vi "GMLAN InitializeConnection.vi"(0 "CAN Interface":string(combo)="CAN1", 5 "Baudrate":u32, 7 "Transmit ID":u32, 9 "Receive ID":u32, 11 "error in (no error)":errorcluster, 12 "UUDT Receive ID":u32) -> (4 "UUDT Engine":T1, 6 "ADCS Ref":T2, 15 "error out":errorcluster)   [LabVIEW 2015, in "GMLAN.lvlib"]
uses:
  GMLAN.lvlib
  <vilib>/Automotive Diagnostic Command Set/Diagnostic Transport.llb/Diag Reference.ctl
  <vilib>/Automotive Diagnostic Command Set/Diagnostic Transport.llb/Transport Protocol Selector.ctl
  <vilib>/Automotive Diagnostic Command Set/Diagnostic Transport.llb/Diag CAN Frame Log.ctl
  _SubVIs/UUDT Engine Refs.ctl
  _SubVIs/UUDT Engine Connection List_Action.ctl
  <vilib>/xnet/xnet.llb/XNET Create Session (Frame Input Queued).vi
  <vilib>/addons/Automotive Diagnostic Command Set/NI_Automotive Diagnostic Command Set.lvlib
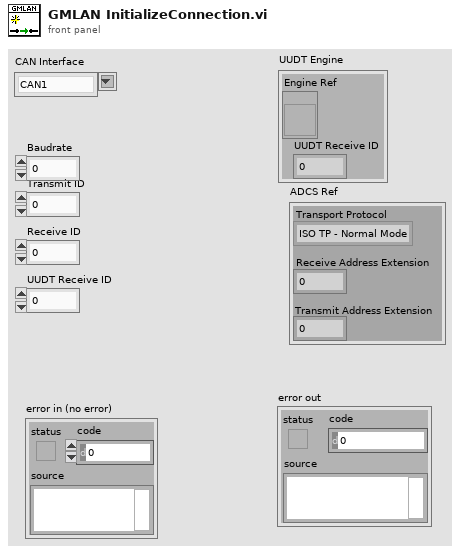
[diagram p1: front panel]
types:
  T1 = typedef "GMLAN.lvlib/UUDT Engine Refs.ctl" = cluster{"Engine Ref":refnum<vi>, "UUDT Receive ID":u32}
  T2 = typedef "NI_Automotive Diagnostic Command Set.lvlib/Diag Reference.ctl" = cluster{"Diag CAN Handle":u32, "Transport Protocol":T3, "Receive Address Extension":u8, "Transmit Address Extension":u8, "Receive CAN Id":u32, "Transmit CAN Id":u32, "Diag CAN Queue":refnum<queue>, "Log Frames ?":bool, "My TP Address":u8, "Other TP Address":u8, "T1":u16, "T2":u16, "T3":u16, "T4":u16, "Tx SN":u8, "Block Size":u8, "Rx SN":u8, "VW TP Initialized?":bool, "Tx block no":u8, "baud rate":u32, "Interface":string, "Channel Diag CAN Handle":u32, "UDP Connection ID":refnum<k16>, "TCP Connection ID":refnum<k5>, "Target IP Addr":u32, "Source Address":u16, "Target Address":u16, "Send Header NACK?":bool, "DLL Handle":u32, "NAD":u8, "Time Stamp read first":dbl, "Time Stamp read last":dbl, "Time Stamp write first":dbl, "Time Stamp write last":dbl, "Time Stamp write":dbl, "Time Stamp read":dbl}
  T3 = typedef "NI_Automotive Diagnostic Command Set.lvlib/Transport Protocol Selector.ctl" = enum16{"ISO TP - Normal Mode", "ISO TP - Mixed Mode", "VW TP 2.0", "Diagnostics on IP", "ISO TP LIN"}
  T4 = typedef "GMLAN.lvlib/UUDT Engine Connection List_Action.ctl" = enum8{"Initialize", "Write", "Add", "Read"}
  T5 = cluster{"Parameter Name":string, "Initial Settings":variant}
  T6 = cluster{"Frame name":string, "Identifier":u32, "Payload Length":u32, "Timing Type":u32, "Transmit Time":dbl, "Extended Identifier?":bool, "Comment":string}
  T7 = cluster{"Parameter Name":string, "Initial Settings":variant}[]
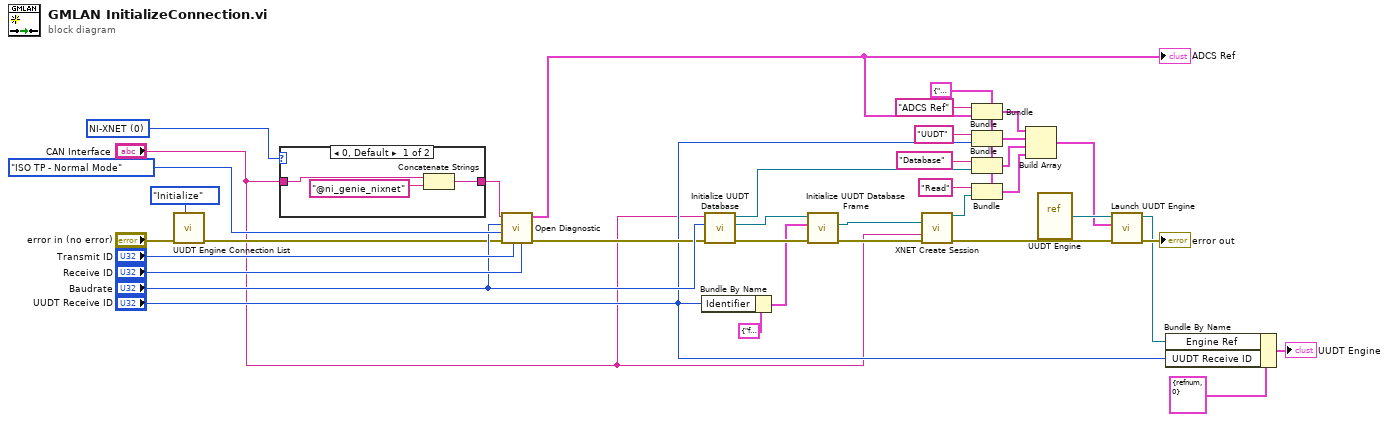
[diagram p0: block diagram]
diagram:
  w3 = u16 0 items=["NI-XNET", "NI-CAN"] ("HW select")
  w18 = T5 {"Parameter Name"="", "Initial Settings"=variant} ("Parameters")
  n1 = call "UUDT Engine Connection List.vi"("Action"=UUDT_Engine_Connection_List_Action."Initialize", "error in"="error in (no error)") -> ("error out"=w5:errorcluster)  [unwired: 8 in, 1 out]
  n2 = case shown="0, Default" w3 {
    tunnel: "CAN Interface" -> [w40 w41]
    tunnel: [w39 w41] -> w1
    frame 0, Default {
      n3 = Concatenate Strings(w40, "@ni_genie_nixnet" ("string")) -> (w39:string)
    }
    frame 1 {
    }
  }
  n4 = call <vilib>:"Open Diagnostic.vi"("Receive ID"="Receive ID", "Transmit ID"="Transmit ID", "error in (no error)"=w5, "Transport Protocol"=Transport_Protocol_Selector."ISO TP - Normal Mode", "Baud Rate"="Baudrate", "CAN Interface"=w1) -> ("error out"=w27:errorcluster, "diag ref out"=w17:T2)  [unwired: 4 out]
  "ADCS Ref" <- w17
  n5 = Bundle By Name(cluster=T6 {"Frame name"="frame1", "Identifier"=1, "Payload Length"=8, "Timing Type"=1, "Transmit Time"=0.0, "Extended Identifier?"=FALSE, "Comment"=""} ("CAN Frame"), "Identifier"="UUDT Receive ID") -> (w29:T6)
  n6 = call "Initialize UUDT Database.vi"("error in (no error)"=w27, "Baud Rate"="Baudrate", "Addon Name"="CAN Interface") -> ("error out"=w34:errorcluster, "Cluster"=w33:refnum<k21>, "XNET Database"=w19:refnum<k21>)  [unwired: 6 in]
  n7 = call "Initialize UUDT Database Frame.vi"("error in"=w34, "CAN Frame"=w29, "cluster in"=w33) -> ("error out"=w31:errorcluster, "frame out"=w32:refnum<k21>)  [unwired: 6 in, 1 out]
  n8 = call-poly <vilib>:"XNET Create Session.vi"("frame"=w32, "interface"="CAN Interface", "error in (no error)"=w31) -> ("session out"=w21:refnum<k21>, "error out"=w26:errorcluster)  [unwired: 11 out]
  n9 = Bundle(cluster=w18, "Parameter Name"="ADCS Ref", "Initial Settings"=w17) -> (w15:T5)
  n10 = Bundle(cluster=w18, "Parameter Name"="UUDT", "Initial Settings"="UUDT Receive ID") -> (w14:T5)
  n11 = Bundle(cluster=w18, "Parameter Name"="Database", "Initial Settings"=w19) -> (w13:T5)
  n12 = Bundle(cluster=w18, "Parameter Name"="Read", "Initial Settings"=w21) -> (w12:T5)
  n13 = Build Array(w15, w14, w13, w12) -> (w11:T7)
  n14 = vi-ref "UUDT Engine.vi"() -> (w24:refnum<vi>)
  n15 = call "Launch UUDT Engine.vi"("error in (no error)"=w26, "Initial Parameters"=w11, "VI Ref In"=w24) -> ("error out"=→"error out":errorcluster, "VI Ref Out"=w10:refnum<vi>)  [unwired: 7 in]
  n16 = Bundle By Name(cluster=T1 {"Engine Ref"=refnum, "UUDT Receive ID"=0} ("UUDT Engine"), "Engine Ref"=w10, "UUDT Receive ID"="UUDT Receive ID") -> (→"UUDT Engine":T1)
